vi "RunScript.vi"(8 "error in":errorcluster, 10 "script":string, 11 "Python":T1) -> (0 "error out":errorcluster, 2 "Tx":string, 3 "Python":T1)   [LabVIEW 2022 SP3]
uses:
  PythonCtrl.ctl
  Processors.ctl
panel:
  out "Reply":string
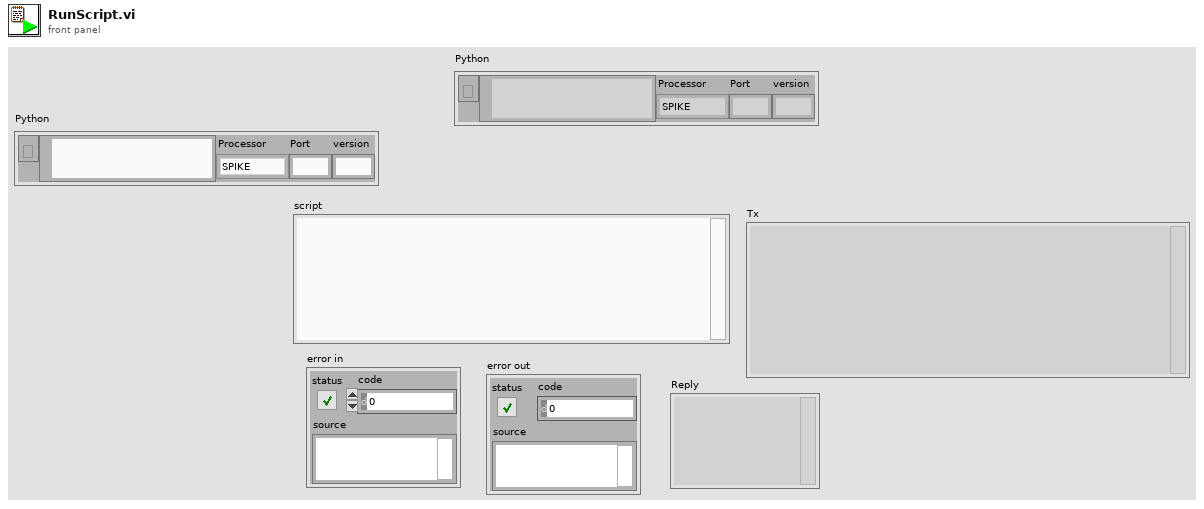
[diagram p1: front panel]
types:
  T1 = typedef "PythonCtrl.ctl" = cluster{"session":refnum<k35>, "PyPath":path, "Processor":T2, "Port":string, "version":string}
  T2 = typedef "Processors.ctl" = enum16{"SPIKE", "Pi", "Pi_ssh", "OpenMV", "Dunio"}
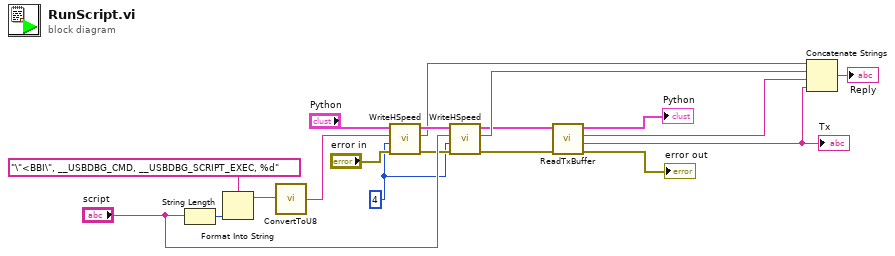
[diagram p0: block diagram]
diagram:
  w1 = 4 ("Reply length")
  n1 = String Length(string="script") -> (length=w18:i32)
  n2 = Format Into String(format string="\"<BBI\", __USBDBG_CMD, __USBDBG_SCRIPT_EXEC, %d" ("write buffer"), w18) -> (resulting string=w7:string)  [unwired: 2 in, 1 out]
  n3 = call "ConvertToU8.vi"("struct"=w7) -> ("Binary"=w6:string)
  n4 = call "WriteHSpeed.vi"("error in"="error in", "Reply length"=w1, "write buffer"=w6, "Python"="Python") -> ("error out"=w14:errorcluster, "read buffer"=w12:string, "Python"=w17:T1)  [unwired: 5 in]
  n5 = call "WriteHSpeed.vi"("error in"=w14, "Reply length"=w1, "write buffer"="script", "Python"=w17) -> ("error out"=w4:errorcluster, "read buffer"=w13:string, "Python"=w3:T1)  [unwired: 5 in]
  n6 = call "ReadTxBuffer.vi"("error in"=w4, "Python"=w3) -> ("error out"=→"error out":errorcluster, "Tx Buffer"=w5:string, "Tx Buffer Len"=w10:string, "Python"=→"Python":T1)  [unwired: 6 in]
  "Tx" <- w5
  n7 = Concatenate Strings(w12, w13, w10, w5) -> (→"Reply":string)
